vi "Config Read Interface.vi"(8 "error in (no error)":errorcluster, 10 "Device Ref in":T1 format="%.0x", 11 "Refnum in":T2) -> (0 "error out":errorcluster, 2 "Device Ref out":T1 format="%.0x", 3 "Refnum out":T2)   [LabVIEW 2021, in "Modbus Master System Explorer.lvlib"]
uses:
  Modbus Master System Explorer.lvlib
  <vilib>/Utility/config.llb/Config Data RefNum.ctl
  <vilib>/NI VeriStand/Custom Device API/Custom Device Item Ref.ctl
  <vilib>/Utility/config.llb/NI_LVConfig.lvlib
  <vilib>/NI VeriStand/Custom Device API/Custom Device API.lvlib
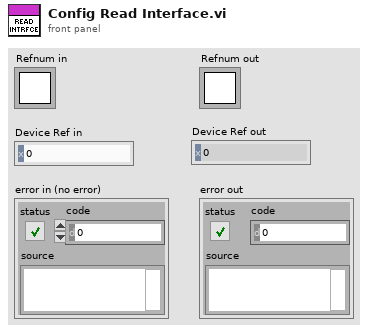
[diagram p1: front panel]
types:
  T1 = typedef "Custom Device API.lvlib/Custom Device Item Ref.ctl" = u64
  T2 = typedef "NI_LVConfig.lvlib/Config Data RefNum.ctl" = refnum<k1>
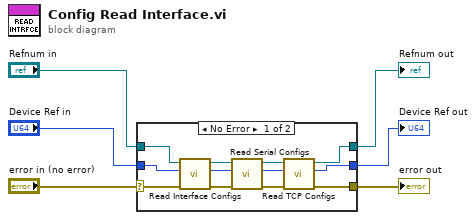
[diagram p0: block diagram]
diagram:
  n1 = case shown="No Error" "error in (no error)" {
    selector: "error in (no error)" -> [w10 w19]
    tunnel: [w15 w21] -> w6
    tunnel: [w13 w19] -> w5
    tunnel: "Refnum in" -> [w9 w21]
    tunnel: [w8 w20] -> w2
    tunnel: "Device Ref in" -> [w7 w20]
    frame No Error {
      n2 = call "Read Interface Configs.vi"("error in (no error)"=w10, "Device Ref in"=w7, "Refnum in"=w9) -> ("error out"=w12:errorcluster, "Item Ref out"=w17:T1, "Refnum out"=w11:T2)  [unwired: 6 in]
      n3 = call "Read Serial Configs.vi"("error in (no error)"=w12, "Item Ref in"=w17, "Refnum in"=w11) -> ("error out"=w14:errorcluster, "Item Ref out"=w16:T1, "Refnum out"=w18:T2)  [unwired: 6 in]
      n4 = call "Read TCP Configs.vi"("error in (no error)"=w14, "Item Ref in"=w16, "Refnum in"=w18) -> ("error out"=w13:errorcluster, "Item Ref out"=w8:T1, "Refnum out"=w15:T2)  [unwired: 6 in]
    }
    frame Error {
    }
  }
  "Refnum out" <- w6
  "error out" <- w5
  "Device Ref out" <- w2
